vi "log analysis_gps.vi"() -> ()   [LabVIEW 2019] (continued)
,0.3081,0.6694,0.1254,0.0948,0.0826,0.1629,0.1651,5.0479,0f000001,0*dfc03d63\n\t", "INSPVAXA,USB3,0,48.5,FINESTEERING,2107,281764.150,02000000,471d,15824;INS_ALIGNMENT_COMPLETE,INS_RTKFIXED,37.37122080817,126.72272865797,8.0273,22.3000,-0.0183,0.2610,0.0199,-0.883754251,-0.497263643,91.594297223,0.5508,0.3085,0.6797,0.1258,0.0948,0.0829,0.1629,0.1651,5.0491,0f000001,0*98c9c36a\n\t", "INSPVAXA,USB3,0,48.5,FINESTEERING,2107,281764.650,02000000,471d,15824;INS_ALIGNMENT_COMPLETE,INS_RTKFIXED,37.37122075325,126.72273024996,8.0307,22.3000,-0.0230,0.2873,0.0155,-0.910536369,-0.571169391,91.698573448,0.5508,0.3085,0.6797,0.1258,0.0948,0.0829,0.1629,0.1651,5.0491,0f000001,0*a48c0ed7\n\t", "INSPVAXA,USB3,0,49.5,FINESTEERING,2107,281765.150,02000000,471d,15824;INS_ALIGNMENT_COMPLETE,INS_RTKFIXED,37.37122068841,126.72273183543,8.0343,22.3000,-0.0165,0.2820,0.0133,-0.835088790,-0.555071717,91.791979713,0.5558,0.3086,0.6882,0.1257,0.0948,0.0832,0.1628,0.1650,5.0496,0f000001,0*cba52910\n\t", "INSPVAXA,USB3,0,49.5,FINESTEERING,2107,281765.650,02000000,471d,15824;INS_ALIGNMENT_COMPLETE,INS_RTKFIXED,37.37122061486,126.72273346284,8.0365,22.3000,-0.0171,0.2746,0.0152,-0.832834423,-0.571575823,91.924169920,0.5558,0.3086,0.6882,0.1257,0.0948,0.0832,0.1628,0.1650,5.0496,0f000001,0*526b2e24\n\t", "INSPVAXA,USB3,0,49.0,FINESTEERING,2107,281766.150,02000000,471d,15824;INS_ALIGNMENT_COMPLETE,INS_RTKFIXED,37.37122054097,126.72273507488,8.0385,22.3000,-0.0218,0.2706,0.0128,-1.000637631,-0.672076774,92.055365430,0.5592,0.3087,0.6949,0.1259,0.0948,0.0833,0.1628,0.1650,5.0498,0f000001,0*57bf3361\n\t", "INSPVAXA,USB3,0,49.0,FINESTEERING,2107,281766.650,02000000,471d,15824;INS_ALIGNMENT_COMPLETE,INS_RTKFIXED,37.37122044479,126.72273670968,8.0412,22.3000,-0.0285,0.2846,0.0116,-1.092573740,-0.740242490,92.171373793,0.5592,0.3087,0.6949,0.1259,0.0948,0.0833,0.1628,0.1650,5.0498,0f000001,0*1c223ea9\n\t", "INSPVAXA,USB3,0,48.0,FINESTEERING,2107,281767.150,02000000,471d,15824;INS_ALIGNMENT_COMPLETE,INS_RTKFIXED,37.37122033445,126.72273829026,8.0449,22.3000,-0.0305,0.2613,0.0217,-0.977094539,-0.639903649,92.271203612,0.5614,0.3086,0.7003,0.1258,0.0947,0.0834,0.1628,0.1649,5.0495,0f000001,0*5c3b8fb1\n\t", "INSPVAXA,USB3,0,48.0,FINESTEERING,2107,281767.650,02000000,471d,15824;INS_ALIGNMENT_COMPLETE,INS_RTKFIXED,37.37122021827,126.72273994335,8.0476,22.3000,-0.0288,0.2733,0.0197,-0.964628632,-0.656119186,92.463441538,0.5614,0.3086,0.7003,0.1258,0.0947,0.0834,0.1628,0.1649,5.0495,0f000001,0*cc7927eb\n\t", "INSPVAXA,USB3,0,48.0,FINESTEERING,2107,281768.150,02000000,471d,15824;INS_ALIGNMENT_COMPLETE,INS_RTKFIXED,37.37122009872,126.72274157958,8.0500,22.3000,-0.0294,0.2847,0.0191,-0.946431620,-0.566462229,92.660906936,0.5627,0.3085,0.7043,0.1259,0.0947,0.0835,0.1628,0.1649,5.0496,0f000001,0*cc13fb9d\n\t", "INSPVAXA,USB3,0,49.0,FINESTEERING,2107,281768.650,02000000,471d,15824;INS_ALIGNMENT_COMPLETE,INS_RTKFIXED,37.37121997801,126.72274320142,8.0509,22.3000,-0.0214,0.2856,0.0260,-1.015543433,-0.231279609,92.847402266,0.5627,0.3085,0.7043,0.1259,0.0947,0.0835,0.1628,0.1649,5.0496,0f000001,0*22053697\n\t", "INSPVAXA,USB3,0,46.5,FINESTEERING,2107,281769.650,02000000,471d,15824;INS_ALIGNMENT_COMPLETE,INS_RTKFIXED,37.37121967893,126.72274645196,8.0567,22.3000,-0.0370,0.2793,0.0333,-0.818626182,0.216920532,93.214992796,0.5635,0.3085,0.7075,0.1258,0.0947,0.0835,0.1628,0.1649,5.0499,0f000001,0*792e5a9d\n\t", "INSPVAXA,USB3,0,48.5,FINESTEERING,2107,281771.150,02000000,471d,15824;INS_ALIGNMENT_COMPLETE,INS_RTKFIXED,37.37121916335,126.72275134411,8.0669,22.3000,-0.0460,0.2833,0.0183,-0.792418480,0.032350312,93.864070762,0.5648,0.3085,0.7116,0.1262,0.0947,0.0836,0.1628,0.1649,5.0523,0f000001,0*03020e62\n\t", "INSPVAXA,USB3,0,47.0,FINESTEERING,2107,281772.150,02000000,471d,15824;INS_ALIGNMENT_COMPLETE,INS_RTKFIXED,37.37121879734,126.72275457125,8.0729,22.3000,-0.0562,0.2927,0.0149,-0.701118394,-0.215535385,94.262257179,0.5652,0.3086,0.7131,0.1264,0.0948,0.0837,0.1628,0.1649,5.0539,0f000001,0*6742cf9b\n\t", "INSPVAXA,USB3,0,47.5,FINESTEERING,2107,281773.150,02000000,471d,15824;INS_ALIGNMENT_COMPLETE,INS_RTKFIXED,37.37121842061,126.72275777876,8.0764,22.3000,-0.0402,0.2880,0.0117,-0.782099339,-0.380092330,94.588227053,0.5655,0.3117,0.7220,0.1266,0.0954,0.0843,0.1628,0.1649,5.0554,0f000001,0*2c781ada\n\t", "INSPVAXA,USB3,0,47.5,FINESTEERING,2107,281774.650,02000000,471d,15824;INS_ALIGNMENT_COMPLETE,INS_RTKFIXED,37.37121790104,126.72276172821,8.0844,22.3000,-0.0056,-0.1159,0.0265,-0.829469010,-1.054819962,94.805665616,0.5657,0.3125,0.7262,0.1269,0.0954,0.0845,0.1628,0.1649,5.0568,0f000001,0*5083390f\n\t", "INSPVAXA,USB3,0,45.5,FINESTEERING,2107,281775.650,02000000,471d,15824;INS_ALIGNMENT_COMPLETE,INS_RTKFIXED,37.37121775993,126.72276174880,8.0908,22.3000,-0.0341,0.2302,0.0228,-0.820870768,-0.784541706,94.618919565,0.5657,0.3121,0.7276,0.1285,0.0952,0.0845,0.1627,0.1649,5.0580,0f000001,0*ef5961e6\n\t", "INSPVAXA,USB3,0,49.5,FINESTEERING,2107,281777.150,02000000,471d,15824;INS_ALIGNMENT_COMPLETE,INS_RTKFIXED,37.37121742515,126.72276471335,8.0933,22.3000,-0.0434,0.3635,0.0199,-0.788823341,-1.034155621,94.704274658,0.5667,0.3105,0.7263,0.1288,0.0950,0.0844,0.1627,0.1648,5.0605,0f000001,0*58cfd0fe\n\t", "INSPVAXA,USB3,0,49.5,FINESTEERING,2107,281780.650,02000000,471d,15824;INS_ALIGNMENT_COMPLETE,INS_RTKFIXED,37.37121639807,126.72277573033,8.0654,22.3000,-0.0075,0.2871,0.0244,-0.701767133,-0.824742936,91.476878975,0.4298,0.3000,0.6003,0.1163,0.0939,0.0789,0.1625,0.1636,5.0634,0f000001,0*3e81e8f3\n\t", "INSPVAXA,USB3,0,49.0,FINESTEERING,2107,281782.150,02000000,471d,15824;INS_ALIGNMENT_COMPLETE,INS_RTKFIXED,37.37121614895,126.72278060077,8.0494,22.3000,-0.0125,0.2941,0.0170,-0.958151284,-0.907972358,90.050842278,0.4192,0.2995,0.5761,0.1162,0.0938,0.0788,0.1624,0.1635,5.0656,0f000001,0*79d70d48\n\t", "INSPVAXA,USB3,0,48.0,FINESTEERING,2107,281794.200,02000000,471d,15824;INS_ALIGNMENT_COMPLETE,INS_RTKFIXED,37.37121538500,126.72279353221,7.9323,22.3000,0.0019,0.0033,0.0055,-1.472038191,-1.222257427,90.266116104,0.2743,0.1995,0.4008,0.0352,0.0349,0.0325,0.1516,0.1495,5.0388,0f000005,0*12f5b6da\n\t", "INSPVAXA,USB3,0,48.0,FINESTEERING,2107,281796.200,02000000,471d,15824;INS_ALIGNMENT_COMPLETE,INS_RTKFIXED,37.37121541125,126.72279352515,7.9254,22.3000,-0.0002,0.0035,0.0060,-1.463145311,-1.218768654,90.268956721,0.2548,0.1854,0.3737,0.0345,0.0343,0.0314,0.1516,0.1493,5.0350,0f000005,0*63f626df\n\t", "INSPVAXA,USB3,0,43.0,FINESTEERING,2107,281797.700,02000000,471d,15824;INS_ALIGNMENT_COMPLETE,INS_RTKFIXED,37.37121541556,126.72279591257,7.9222,22.3000,-0.0052,0.3417,0.0085,-1.766936692,-1.171645490,90.396175106,0.2469,0.1802,0.3627,0.0345,0.0343,0.0313,0.1515,0.1492,5.0303,0f000005,0*2970234a\n\t", "INSPVAXA,USB3,0,45.5,FINESTEERING,2107,281798.700,02000000,471d,15824;INS_ALIGNMENT_COMPLETE,INS_RTKFIXED,37.37121535057,126.72279879079,7.9235,22.3000,-0.0085,0.3000,0.0138,-1.696631834,-1.054944377,90.699133923,0.2423,0.1802,0.3574,0.0527,0.0471,0.0400,0.1536,0.1513,5.0319,0f000001,0*b28cf3b5\n\t", "INSPVAXA,USB3,0,46.0,FINESTEERING,2107,281800.200,02000000,471d,15824;INS_ALIGNMENT_COMPLETE,INS_RTKFIXED,37.37121518346,126.72280384244,7.9320,22.3000,-0.0138,0.3041,-0.0020,-1.831014383,-0.921017115,91.358421751,0.2498,0.2023,0.3609,0.0772,0.0698,0.0531,0.1576,0.1555,5.0235,0f000001,0*fd249ab4\n\t", "INSPVAXA,USB3,0,45.0,FINESTEERING,2107,281801.700,02008000,471d,15824;INS_ALIGNMENT_COMPLETE,INS_RTKFIXED,37.37121487597,126.72280876147,7.9415,22.3000,-0.0281,0.2809,0.0050,-1.870107911,-0.684128774,92.617548886,0.2701,0.2229,0.3702,0.0875,0.0787,0.0583,0.1591,0.1573,5.0044,0f000001,0*b89165ad\n\t", "INSPVAXA,USB3,0,48.0,FINESTEERING,2107,281802.700,02008000,471d,15824;INS_ALIGNMENT_COMPLETE,INS_RTKFIXED,37.37121453908,126.72281198538,7.9511,22.3000,-0.0315,0.2792,0.0111,-1.788436181,-0.484915836,93.932977011,0.2978,0.2449,0.3840,0.0951,0.0852,0.0628,0.1602,0.1589,4.9745,0f000001,0*1b429bef\n\t", "INSPVAXA,USB3,0,48.5,FINESTEERING,2107,281804.200,02008000,471d,15824;INS_ALIGNMENT_COMPLETE,INS_RTKFIXED,37.37121383035,126.72281674518,7.9651,22.3000,-0.0315,0.2774,0.0174,-1.651879586,-0.284385340,95.400888665,0.3536,0.2781,0.4212,0.1050,0.0912,0.0696,0.1611,0.1606,4.9104,0f000001,0*27f05722\n\t", "INSPVAXA,USB3,0,48.5,FINESTEERING,2107,281804.700,02008000,471d,15824;INS_ALIGNMENT_COMPLETE,INS_RTKFIXED,37.37121355118,126.72281832287,7.9691,22.3000,-0.0490,0.2623,0.0114,-1.600367868,-0.284854057,95.675635132,0.3536,0.2781,0.4212,0.1050,0.0912,0.0696,0.1611,0.1606,4.9104,0f000001,0*fdce50cc\n\t", "INSPVAXA,USB3,0,47.5,FINESTEERING,2107,281806.200,02000000,471d,15824;INS_ALIGNMENT_COMPLETE,INS_RTKFIXED,37.37121269576,126.72282281458,7.9853,22.3000,-0.0549,0.2699,0.0235,-1.099815041,-0.190468307,96.163961880,0.3893,0.2926,0.4618,0.1082,0.0921,0.0739,0.1610,0.1610,4.8764,0f000001,0*3796a6d3\n\t", "INSPVAXA,USB3,0,49.0,FINESTEERING,2107,281807.200,02000000,471d,15824;INS_ALIGNMENT_COMPLETE,INS_RTKFIXED,37.37121211278,126.72282605036,7.9969,22.3000,-0.0568,0.3027,0.0138,-1.053067803,-0.177291074,96.270087858,0.3995,0.2955,0.4805,0.1085,0.0920,0.0753,0.1609,0.1610,4.8712,0f000001,0*6bce3c8a\n\t", "INSPVAXA,USB3,0,49.0,FINESTEERING,2107,281807.700,02000000,471d,15824;INS_ALIGNMENT_COMPLETE,INS_RTKFIXED,37.37121182995,126.72282768938,8.0018,22.3000,-0.0581,0.2574,0.0176,-1.058374656,-0.238658340,96.102791514,0.3995,0.2955,0.4805,0.1085,0.0920,0.0753,0.1609,0.1610,4.8712,0f000001,0*be10ea19\n\t", "INSPVAXA,USB3,0,50.0,FINESTEERING,2107,281808.200,02000000,471d,15824;INS_ALIGNMENT_COMPLETE,INS_RTKFIXED,37.37121156109,126.72282925658,8.0066,22.3000,-0.0729,0.2643,0.0186,-0.872363263,-0.172820983,95.527165768,0.4058,0.2969,0.4970,0.1085,0.0920,0.0762,0.1608,0.1609,4.8702,0f000001,0*2e1aa4d5\n\t", "INSPVAXA,USB3,0,47.5,FINESTEERING,2107,281810.700,02000000,471d,15824;INS_ALIGNMENT_COMPLETE,INS_RTKFIXED,37.37121067103,126.72283703860,8.0191,22.3000,-0.0356,0.2756,0.0276,-0.647693750,-0.582187036,89.865016518,0.4124,0.2979,0.5229,0.1081,0.0920,0.0770,0.1607,0.1609,4.8726,0f000001,0*855b65fe\n\t", "INSPVAXA,USB3,0,45.5,FINESTEERING,2107,281811.200,02000000,471d,15824;INS_ALIGNMENT_COMPLETE,INS_RTKFIXED,37.37121058449,126.72283863071,8.0196,22.3000,-0.0335,0.2776,0.0134,-0.642436462,-0.620062849,88.791539404,0.4132,0.2980,0.5319,0.1079,0.0921,0.0771,0.1607,0.1609,4.8738,0f000001,0*5d2242c7\n\t", "INSPVAXA,USB3,0,45.5,FINESTEERING,2107,281811.700,02000000,471d,15824;INS_ALIGNMENT_COMPLETE,INS_RTKFIXED,37.37121052303,126.72284024830,8.0190,22.3000,-0.0385,0.2808,0.0125,-0.613070377,-0.534497293,88.053265281,0.4132,0.2980,0.5319,0.1079,0.0921,0.0771,0.1607,0.1609,4.8738,0f000001,0*21e07958\n\t", "INSPVAXA,USB3,0,48.5,FINESTEERING,2107,281812.200,02000000,471d,15824;INS_ALIGNMENT_COMPLETE,INS_RTKFIXED,37.37121047493,126.72284184822,8.0183,22.3000,-0.0314,0.2883,0.0148,-0.539418931,-0.410155130,87.563487932,0.4135,0.2980,0.5387,0.1083,0.0923,0.0770,0.1607,0.1609,4.8744,0f000001,0*aee609c3\n\t", "INSPVAXA,USB3,0,48.5,FINESTEERING,2107,281812.700,02000000,471d,15824;INS_ALIGNMENT_COMPLETE,INS_RTKFIXED,37.37121044769,126.72284347413,8.0176,22.3000,-0.0247,0.2718,0.0203,-0.569551057,-0.519035178,87.323829382,0.4135,0.2980,0.5387,0.1083,0.0923,0.0770,0.1607,0.1609,4.8744,0f000001,0*0b29fab3\n\t", "INSPVAXA,USB3,0,49.5,FINESTEERING,2107,281813.200,02000000,471d,15824;INS_ALIGNMENT_COMPLETE,INS_RTKFIXED,37.37121043009,126.72284509802,8.0163,22.3000,-0.0270,0.2716,0.0250,-0.708149800,-0.786508619,87.284677212,0.4137,0.2982,0.5437,0.1082,0.0926,0.0769,0.1607,0.1609,4.8743,0f000001,0*3e525f31\n\t", "INSPVAXA,USB3,0,49.5,FINESTEERING,2107,281813.700,02000000,471d,15824;INS_ALIGNMENT_COMPLETE,INS_RTKFIXED,37.37121041419,126.72284671710,8.0139,22.3000,-0.0269,0.2730,0.0206,-0.734434421,-0.847262919,87.384621044,0.4137,0.2982,0.5437,0.1082,0.0926,0.0769,0.1607,0.1609,4.8743,0f000001,0*ad1d52fd\n\t", "INSPVAXA,USB3,0,51.5,FINESTEERING,2107,281814.200,02000000,471d,15824;INS_ALIGNMENT_COMPLETE,INS_RTKFIXED,37.37121039679,126.72284831835,8.0121,22.3000,-0.0282,0.2780,0.0157,-0.723695017,-0.718771223,87.478292195,0.4133,0.2982,0.5471,0.1087,0.0929,0.0768,0.1607,0.1609,4.8744,0f000001,0*2471b93a\n\t", "INSPVAXA,USB3,0,51.5,FINESTEERING,2107,281814.700,02000000,471d,15824;INS_ALIGNMENT_COMPLETE,INS_RTKFIXED,37.37121037596,126.72284994702,8.0093,22.3000,-0.0392,0.2745,0.0084,-0.653618450,-0.794919707,87.628354192,0.4133,0.2982,0.5471,0.1087,0.0929,0.0768,0.1607,0.1609,4.8744,0f000001,0*e403a187\n\t", "INSPVAXA,USB3,0,48.5,FINESTEERING,2107,281815.200,02000000,471d,15824;INS_ALIGNMENT_COMPLETE,INS_RTKFIXED,37.37121035462,126.72285153134,8.0061,22.3000,-0.0298,0.2645,0.0056,-0.689462144,-0.765571273,87.819585359,0.4135,0.2983,0.5496,0.1092,0.0931,0.0767,0.1607,0.1609,4.8745,0f000001,0*3d6e9c36\n\t", "INSPVAXA,USB3,0,48.5,FINESTEERING,2107,281815.700,02000000,471d,15824;INS_ALIGNMENT_COMPLETE,INS_RTKFIXED,37.37121033500,126.72285311005,8.0032,22.3000,-0.0264,0.2987,0.0158,-0.781716650,-0.583090906,88.033249941,0.4135,0.2983,0.5496,0.1092,0.0931,0.0767,0.1607,0.1609,4.8745,0f000001,0*4dfcf1d6\n\t", "INSPVAXA,USB3,0,51.0,FINESTEERING,2107,281816.200,02008000,471d,15824;INS_ALIGNMENT_COMPLETE,INS_RTKFIXED,37.37121030517,126.72285487145,8.0002,22.3000,-0.0425,0.2860,0.0120,-0.722434536,-0.707507472,88.283028579,0.4136,0.2984,0.5510,0.1094,0.0933,0.0766,0.1607,0.1609,4.8747,0f000001,0*7939fe65\n\t", "INSPVAXA,USB3,0,51.0,FINESTEERING,2107,281816.700,02008000,471d,15824;INS_ALIGNMENT_COMPLETE,INS_RTKFIXED,37.37121027801,126.72285655609,7.9980,22.3000,-0.0398,0.3098,0.0245,-0.754705884,-0.828367575,88.621683950,0.4136,0.2984,0.5510,0.1094,0.0933,0.0766,0.1607,0.1609,4.8747,0f000001,0*590aa229\n\t", "INSPVAXA,USB3,0,48.5,FINESTEERING,2107,281817.200,02008000,471d,15824;INS_ALIGNMENT_COMPLETE,INS_RTKFIXED,37.37121021919,126.72285821539,7.9935,22.3000,-0.0399,0.3049,0.0009,-0.558805216,-0.866819508,89.180337786,0.4133,0.2986,0.5518,0.1098,0.0934,0.0766,0.1606,0.1608,4.8755,0f000001,0*c032cfc0\n\t", "INSPVAXA,USB3,0,48.5,FINESTEERING,2107,281817.700,02008000,471d,15824;INS_ALIGNMENT_COMPLETE,INS_RTKFIXED,37.37121014797,126.72285990079,7.9875,22.3000,-0.0366,0.2866,-0.0014,-0.542824992,-1.209169915,90.078081458,0.4133,0.2986,0.5518,0.1098,0.0934,0.0766,0.1606,0.1608,4.8755,0f000001,0*9b0194b0\n\t", "INSPVAXA,USB3,0,48.0,FINESTEERING,2107,281818.200,02008000,471d,15824;INS_ALIGNMENT_COMPLETE,INS_RTKFIXED,37.37121006905,126.72286154850,7.9830,22.3000,-0.0357,0.2838,0.0134,-0.818598247,-1.286018630,91.179102857,0.4133,0.2987,0.5521,0.1099,0.0933,0.0766,0.1606,0.1607,4.8765,0f000001,0*fb948376\n\t", "INSPVAXA,USB3,0,48.0,FINESTEERING,2107,281818.700,02008000,471d,15824;INS_ALIGNMENT_COMPLETE,INS_RTKFIXED,37.37120996329,126.72286319027,7.9792,22.3000,-0.0377,0.2984,0.0070,-0.940731055,-1.250722578,92.396481410,0.4133,0.2987,0.5521,0.1099,0.0933,0.0766,0.1606,0.1607,4.8765,0f000001,0*0f67b83c\n\t", "INSPVAXA,USB3,0,49.0,FINESTEERING,2107,281819.200,02008000,471d,15824;INS_ALIGNMENT_COMPLETE,INS_RTKFIXED,37.37120981052,126.72286484515,7.9750,22.3000,-0.0478,0.2879,0.0099,-0.798984239,-1.444181950,93.568970081,0.4129,0.2987,0.5522,0.1099,0.0932,0.0766,0.1605,0.1605,4.8778,0f000001,0*6b031fe9\n\t", "INSPVAXA,USB3,0,49.0,FINESTEERING,2107,281819.700,02008000,471d,15824;INS_ALIGNMENT_COMPLETE,INS_RTKFIXED,37.37120962300,126.72286650676,7.9705,22.3000,-0.0671,0.2946,0.0135,-0.649128294,-1.472904568,94.664078192,0.4129,0.2987,0.5522,0.1099,0.0932,0.0766,0.1605,0.1605,4.8778,0f000001,0*2bf58c7b\n\t", "INSPVAXA,USB3,0,48.5,FINESTEERING,2107,281820.200,02008000,471d,15824;INS_ALIGNMENT_COMPLETE,INS_RTKFIXED,37.37120940139,126.72286814747,7.9651,22.3000,-0.0641,0.2873,0.0149,-0.504838875,-1.441095327,95.746291084,0.4127,0.2987,0.5521,0.1098,0.0930,0.0766,0.1605,0.1604,4.8792,0f000001,0*7c1d55f3\n\t", "INSPVAXA,USB3,0,48.5,FINESTEERING,2107,281820.700,02008000,471d,15824;INS_ALIGNMENT_COMPLETE,INS_RTKFIXED,37.37120917103,126.72286978921,7.9589,22.3000,-0.0688,0.2879,0.0058,-0.603273984,-1.593663516,96.633630255,0.4127,0.2987,0.5521,0.1098,0.0930,0.0766,0.1605,0.1604,4.8792,0f000001,0*e21ec5f9\n\t", "DUALANTENNAHEADINGA,USB3,0,48.5,FINESTEERING,2107,281821.200,02000000,d426,15824;SOL_COMPUTED,NARROW_FLOAT,-1.000000000,199.802429199,59.611751556,0.0,103.871536255,169.545913696,\"631T\",19,8,8,8,04,00,20,23*e0db817a\n\t", "INSPVAXA,USB3,0,48.5,FINESTEERING,2107,281821.700,02000000,471d,15824;INS_ALIGNMENT_COMPLETE,INS_RTKFIXED,37.37120867107,126.72287305353,7.9486,22.3000,-0.0854,0.2737,-0.0020,-0.718036711,-1.580500229,97.593601208,0.4126,0.2986,0.5520,0.1098,0.0929,0.0766,0.1604,0.1603,4.8804,0f000001,0*a82ce81c\n\t", "INSPVAXA,USB3,0,51.0,FINESTEERING,2107,281822.200,02000000,471d,15824;INS_ALIGNMENT_COMPLETE,INS_RTKFIXED,37.37120839710,126.72287464148,7.9433,22.3000,-0.0737,0.2706,0.0058,-0.493099711,-1.491040971,97.883869188,0.4123,0.2985,0.5518,0.1098,0.0930,0.0767,0.1604,0.1602,4.8814,0f000001,0*43cf4a7f\n\t", "DUALANTENNAHEADINGA,USB3,0,51.0,FINESTEERING,2107,281822.700,02000000,d426,15824;SOL_COMPUTED,NARROW_FLOAT,-1.000000000,199.656448364,63.340484619,0.0,99.066596985,82.183616638,\"631T\",18,8,8,8,04,00,20,23*3eb0b03b\n\t", "INSPVAXA,USB3,0,46.0,FINESTEERING,2107,281823.200,02000000,471d,15824;INS_ALIGNMENT_COMPLETE,INS_RTKFIXED,37.37120785592,126.72287776108,7.9348,22.3000,-0.0813,0.2968,0.0005,-0.426101177,-1.082566624,98.131503900,0.4122,0.2985,0.5517,0.1098,0.0931,0.0768,0.1603,0.1602,4.8821,0f000001,0*e97d0866\n\t", "DUALANTENNAHEADINGA,USB3,0,46.0,FINESTEERING,2107,281823.700,02000000,d426,15824;SOL_COMPUTED,NARROW_FLOAT,-1.000000000,152.081710815,66.315963745,0.0,360.000000000,174.707107544,\"631T\",18,9,9,8,04,00,20,23*2d86097d\n\t", "DUALANTENNAHEADINGA,USB3,0,50.0,FINESTEERING,2107,281824.200,02000000,d426,15824;SOL_COMPUTED,NARROW_FLOAT,-1.000000000,155.447463989,72.039955139,0.0,360.000000000,145.525100708,\"631T\",18,9,9,8,04,00,20,23*f6d7a9cd\n\t", "INSPVAXA,USB3,0,50.0,FINESTEERING,2107,281824.700,02000000,471d,15824;INS_ALIGNMENT_COMPLETE,INS_RTKFIXED,37.37120702523,126.72288248256,7.9286,22.3000,-0.1000,0.2970,-0.0030,-0.414363931,-1.319109492,98.317764432,0.4124,0.2984,0.5515,0.1099,0.0933,0.0768,0.1603,0.1602,4.8829,0f000001,0*6aa4622c\n\t", "DUALANTENNAHEADINGA,USB3,0,49.5,FINESTEERING,2107,281825.200,02000000,d426,15824;SOL_COMPUTED,L1_FLOAT,-1.000000000,69.256408691,12.160554886,0.0,285.962799072,180.000000000,\"631T\",19,8,8,5,04,00,20,21*0683b703\n\t", "INSPVAXA,USB3,0,49.5,FINESTEERING,2107,281825.700,02000000,471d,15824;INS_ALIGNMENT_COMPLETE,INS_RTKFIXED,37.37120646463,126.72288578375,7.9281,22.3000,-0.0763,0.2904,0.0216,-0.793323324,-0.889298592,98.320200190,0.4125,0.2985,0.5514,0.1101,0.0934,0.0769,0.1602,0.1602,4.8839,0f000001,0*5f866581\n\t", "INSPVAXA,USB3,0,48.5,FINESTEERING,2107,281826.200,02000000,471d,15824;INS_ALIGNMENT_COMPLETE,INS_RTKFIXED,37.37120619057,126.72288730405,7.9253,22.3000,-0.0749,0.2848,0.0194,-0.697963338,-0.472482314,97.902378657,0.4129,0.2985,0.5514,0.1102,0.0935,0.0770,0.1601,0.1601,4.8852,0f000001,0*4b4d602c\n\t", "INSPVAXA,USB3,0,48.5,FINESTEERING,2107,281826.700,02000000,471d,15824;INS_ALIGNMENT_COMPLETE,INS_RTKFIXED,37.37120593844,126.72288885558,7.9222,22.3000,-0.0660,0.2989,0.0157,-0.925431746,0.038687863,97.361199599,0.4129,0.2985,0.5514,0.1102,0.0935,0.0770,0.1601,0.1601,4.8852,0f000001,0*d022d5ea\n\t", "DUALANTENNAHEADINGA,USB3,0,49.5,FINESTEERING,2107,281827.200,02000000,d426,15824;SOL_COMPUTED,NARROW_FLOAT,-1.000000000,106.272483826,69.863449097,0.0,360.000000000,180.000000000,\"631T\",18,5,5,5,04,00,20,03*ec53100b\n\t", "INSPVAXA,USB3,0,49.5,FINESTEERING,2107,281827.700,02000000,471d,15824;INS_ALIGNMENT_COMPLETE,INS_RTKFIXED,37.37120552459,126.72289199783,7.9230,22.3000,-0.0613,0.2731,0.0106,-1.441869650,0.390097771,95.831538133,0.4135,0.2986,0.5515,0.1109,0.0937,0.0770,0.1599,0.1601,4.8868,0f000001,0*586a71ed\n\t", "INSPVAXA,USB3,0,51.0,FINESTEERING,2107,281828.200,02000000,471d,15824;INS_ALIGNMENT_COMPLETE,INS_RTKFIXED,37.37120533257,126.72289355096,7.9234,22.3000,-0.0675,0.2814,0.0290,-1.476207155,0.673066178,94.890255810,0.4144,0.2985,0.5514,0.1108,0.0941,0.0770,0.1598,0.1600,4.8875,0f000001,0*65bdbb94\n\t", "INSPVAXA,USB3,0,51.0,FINESTEERING,2107,281828.700,02000000,471d,15824;INS_ALIGNMENT_COMPLETE,INS_RTKFIXED,37.37120515804,126.72289518020,7.9256,22.3000,-0.0694,0.2933,0.0211,-1.265355938,0.544212560,94.152212733,0.4144,0.2985,0.5514,0.1108,0.0941,0.0770,0.1598,0.1600,4.8875,0f000001,0*3fa45f89\n\t", "INSPVAXA,USB3,0,46.5,FINESTEERING,2107,281829.200,02000000,471d,15824;INS_ALIGNMENT_COMPLETE,INS_RTKFIXED,37.37120502580,126.72289678148,7.9278,22.3000,-0.0502,0.2768,0.0145,-1.429978780,0.528599128,93.605134571,0.4154,0.2985,0.5516,0.1105,0.0939,0.0771,0.1597,0.1599,4.8857,0f000001,0*990165b1\n\t", "DUALANTENNAHEADINGA,USB3,0,46.5,FINESTEERING,2107,281829.700,02000000,d426,15824;SOL_COMPUTED,NARROW_FLOAT,-1.000000000,57.886253357,2.555429220,0.0,154.963073730,180.000000000,\"631T\",19,7,7,5,04,00,20,03*f9e0cff3\n\t", "DUALANTENNAHEADINGA,USB3,0,49.5,FINESTEERING,2107,281830.200,02000000,d426,15824;SOL_COMPUTED,L1_FLOAT,-1.000000000,83.986137390,10.132819176,0.0,360.000000000,180.000000000,\"631T\",19,6,6,3,04,00,20,01*1abfa712\n\t", "INSPVAXA,USB3,0,49.5,FINESTEERING,2107,281830.700,02000000,471d,15824;INS_ALIGNMENT_COMPLETE,INS_RTKFIXED,37.37120465229,126.72290157166,7.9350,22.3000,-0.0442,0.2947,0.0242,-1.334244960,0.390910805,92.567102853,0.4155,0.2984,0.5517,0.1101,0.0937,0.0771,0.1595,0.1599,4.8819,0f000001,0*e118fdc5\n\t", "DUALANTENNAHEADINGA,USB3,0,50.0,FINESTEERING,2107,281831.200,02000000,d426,15824;SOL_COMPUTED,NARROW_FLOAT,-1.000000000,59.043685913,-28.864562988,0.0,170.366668701,180.000000000,\"631T\",18,8,8,7,04,00,20,23*14dad2b0\n\t", "DUALANTENNAHEADINGA,USB3,0,50.0,FINESTEERING,2107,281831.700,02000000,d426,15824;SOL_COMPUTED,NARROW_FLOAT,-1.000000000,59.094017029,-28.251525879,0.0,171.144256592,180.000000000,\"631T\",17,8,8,7,04,00,20,23*b1c96c44\n\t", "DUALANTENNAHEADINGA,USB3,0,51.0,FINESTEERING,2107,281832.200,02000000,d426,15824;SOL_COMPUTED,NARROW_FLOAT,-1.000000000,147.351470947,72.022521973,0.0,360.000000000,180.000000000,\"631T\",17,7,7,7,04,00,20,23*e605d7f3\n\t", "DUALANTENNAHEADINGA,USB3,0,51.0,FINESTEERING,2107,281832.700,02000000,d426,15824;SOL_COMPUTED,NARROW_FLOAT,-1.000000000,140.025573730,68.472808838,0.0,360.000000000,180.000000000,\"631T\",16,7,7,7,04,00,20,23*882fbccd\n\t", "DUALANTENNAHEADINGA,USB3,0,50.5,FINESTEERING,2107,281833.200,02000000,d426,15824;SOL_COMPUTED,NARROW_FLOAT,-1.000000000,68.082496643,-11.763427734,0.0,169.499374390,180.000000000,\"631T\",18,9,9,7,04,00,20,23*031ca633\n\t", "DUALANTENNAHEADINGA,USB3,0,50.5,FINESTEERING,2107,281833.700,02000000,d426,15824;SOL_COMPUTED,NARROW_FLOAT,-1.000000000,67.931724548,-11.679229736,0.0,169.789916992,180.000000000,\"631T\",18,9,9,7,04,00,20,23*9183d900\n\t", "DUALANTENNAHEADINGA,USB3,0,47.0,FINESTEERING,2107,281834.200,02000000,d426,15824;SOL_COMPUTED,NARROW_FLOAT,-1.000000000,117.470924377,63.855136871,0.0,360.000000000,180.000000000,\"631T\",18,5,5,5,04,00,20,03*04244261\n\t", "INSPVAXA,USB3,0,47.0,FINESTEERING,2107,281834.700,02000000,471d,15824;INS_ALIGNMENT_COMPLETE,INS_RTKFIXED,37.37120376020,126.72291436834,7.9622,22.3000,-0.0339,0.2802,0.0380,-1.719157085,0.362405119,93.876835430,0.4140,0.2983,0.5521,0.1098,0.0930,0.0772,0.1595,0.1599,4.8699,0f000001,0*4c3c706d\n\t", "DUALANTENNAHEADINGA,USB3,0,49.5,FINESTEERING,2107,281835.200,02000000,d426,15824;SOL_COMPUTED,NARROW_FLOAT,-1.000000000,56.406482697,-13.603881836,0.0,133.707977295,180.000000000,\"631T\",17,6,6,5,04,00,20,03*0c459025\n\t", "DUALANTENNAHEADINGA,USB3,0,49.5,FINESTEERING,2107,281835.700,02000000,d426,15824;SOL_COMPUTED,NARROW_FLOAT,-1.000000000,56.377288818,-12.403900146,0.0,134.026809692,180.000000000,\"631T\",18,6,6,5,04,00,20,03*a9390bed\n\t", "INSPVAXA,USB3,0,49.5,FINESTEERING,2107,281836.200,02000000,471d,15824;INS_ALIGNMENT_COMPLETE,INS_RTKFIXED,37.37120330531,126.72291919762,7.9715,22.3000,-0.0485,0.2910,0.0305,-1.607227145,0.177759790,96.248616069,0.4130,0.2982,0.5522,0.1099,0.0930,0.0773,0.1596,0.1599,4.8709,0f000001,0*7239ccf3\n\t", "DUALANTENNAHEADINGA,USB3,0,49.5,FINESTEERING,2107,281836.700,02000000,d426,15824;SOL_COMPUTED,L1_FLOAT,-1.000000000,75.942611694,16.211278915,0.0,339.522399902,180.000000000,\"631T\",19,6,6,3,04,00,20,01*51b3f26e\n\t", "DUALANTENNAHEADINGA,USB3,0,48.5,FINESTEERING,2107,281837.200,02000000,d426,15824;SOL_COMPUTED,L1_FLOAT,-1.000000000,80.771942139,6.980556488,0.0,360.000000000,180.000000000,\"631T\",20,5,5,2,04,00,20,01*7f238ca7\n\t", "DUALANTENNAHEADINGA,USB3,0,48.5,FINESTEERING,2107,281837.700,02000000,d426,15824;SOL_COMPUTED,L1_FLOAT,-1.000000000,81.947074890,7.586090088,0.0,360.000000000,180.000000000,\"631T\",19,5,5,2,04,00,20,01*fab92539\n\t", "DUALANTENNAHEADINGA,USB3,0,50.5,FINESTEERING,2107,281838.200,02000000,d426,15824;SOL_COMPUTED,NARROW_FLOAT,-1.000000000,70.339691162,-8.337524414,0.0,360.000000000,180.000000000,\"631T\",19,5,5,5,04,00,20,03*774b3c80\n\t", "DUALANTENNAHEADINGA,USB3,0,50.5,FINESTEERING,2107,281838.700,02000000,d426,15824;SOL_COMPUTED,NARROW_FLOAT,-1.000000000,76.530433655,10.538305283,0.0,360.000000000,180.000000000,\"631T\",20,5,5,5,04,00,20,03*8a1753aa\n\t", "DUALANTENNAHEADINGA,USB3,0,48.5,FINESTEERING,2107,281839.200,02000000,d426,15824;SOL_COMPUTED,NARROW_FLOAT,-1.000000000,124.470252991,58.985340118,0.0,360.000000000,180.000000000,\"631T\",20,7,7,7,04,00,20,23*a245761b\n\t", "DUALANTENNAHEADINGA,USB3,0,48.5,FINESTEERING,2107,281839.700,02000000,d426,15824;SOL_COMPUTED,NARROW_FLOAT,-1.000000000,152.317840576,70.615020752,0.0,360.000000000,180.000000000,\"631T\",18,5,5,5,04,00,20,03*7061d411\n\t", "DUALANTENNAHEADINGA,USB3,0,48.0,FINESTEERING,2107,281840.200,02000000,d426,15824;SOL_COMPUTED,L1_FLOAT,-1.000000000,81.231452942,8.750979424,0.0,360.000000000,180.000000000,\"631T\",18,6,6,3,04,00,20,01*4b849010\n\t", "DUALANTENNAHEADINGA,USB3,0,48.0,FINESTEERING,2107,281840.700,02000000,d426,15824;SOL_COMPUTED,L1_FLOAT,-1.000000000,82.520584106,5.924606323,0.0,360.000000000,180.000000000,\"631T\",18,6,6,3,04,00,20,01*b6060555\n\t", "DUALANTENNAHEADINGA,USB3,0,49.0,FINESTEERING,2107,281841.200,02000000,d426,15824;SOL_COMPUTED,L1_FLOAT,-1.000000000,85.243263245,10.185308456,0.0,360.000000000,180.000000000,\"631T\",19,6,6,3,04,00,20,01*39a33d99\n\t", "DUALANTENNAHEADINGA,USB3,0,49.0,FINESTEERING,2107,281841.700,02000000,d426,15824;SOL_COMPUTED,L1_FLOAT,-1.000000000,84.280883789,10.021371841,0.0,360.000000000,180.000000000,\"631T\",20,6,6,3,04,00,20,01*b97d95c9\n\t", "DUALANTENNAHEADINGA,USB3,0,49.5,FINESTEERING,2107,281842.200,02000000,d426,15824;SOL_COMPUTED,NARROW_FLOAT,-1.000000000,70.006813049,-31.901763916,0.0,210.151992798,180.000000000,\"631T\",17,7,7,5,04,00,20,03*5ed3d42a\n\t", "DUALANTENNAHEADINGA,USB3,0,49.5,FINESTEERING,2107,281842.700,02000000,d426,15824;SOL_COMPUTED,NARROW_FLOAT,-1.000000000,69.602676392,-30.153381348,0.0,208.420791626,180.000000000,\"631T\",17,7,7,5,04,00,20,03*0e8eebe2\n\t", "DUALANTENNAHEADINGA,USB3,0,49.5,FINESTEERING,2107,281843.200,02000000,d426,15824;SOL_COMPUTED,NARROW_FLOAT,-1.000000000,134.588546753,49.958206177,0.0,360.000000000,180.000000000,\"631T\",17,5,5,5,04,00,20,03*524a8851\n\t", "DUALANTENNAHEADINGA,USB3,0,49.5,FINESTEERING,2107,281843.700,02000000,d426,15824;SOL_COMPUTED,NARROW_FLOAT,-1.000000000,111.024063110,4.724229813,0.0,360.000000000,180.000000000,\"631T\",17,5,5,5,04,00,20,03*868053f4\n\t", "DUALANTENNAHEADINGA,USB3,0,50.0,FINESTEERING,2107,281844.200,02000000,d426,15824;SOL_COMPUTED,L1_FLOAT,-1.000000000,91.707588196,-1.773010254,0.0,360.000000000,180.000000000,\"631T\",17,6,6,3,04,00,20,01*2b557997\n\t", "DUALANTENNAHEADINGA,USB3,0,50.0,FINESTEERING,2107,281845.700,02000000,d426,15824;SOL_COMPUTED,NARROW_FLOAT,-1.000000000,48.226726532,-51.942321777,0.0,56.526073456,74.567710876,\"631T\",21,6,6,5,04,00,20,03*278cdd49\n\t", "DUALANTENNAHEADINGA,USB3,0,50.0,FINESTEERING,2107,281846.200,02000000,d426,15824;SOL_COMPUTED,L1_FLOAT,-1.000000000,98.548431396,11.085563660,0.0,360.000000000,180.000000000,\"631T\",20,6,6,3,04,00,20,01*4cd03511\n\t", "DUALANTENNAHEADINGA,USB3,0,50.0,FINESTEERING,2107,281846.700,02000000,d426,15824;SOL_COMPUTED,L1_FLOAT,-1.000000000,97.773071289,12.519289017,0.0,360.000000000,180.000000000,\"631T\",20,6,6,3,04,00,20,01*fc76e214\n\t", "DUALANTENNAHEADINGA,USB3,0,48.5,FINESTEERING,2107,281847.200,02000000,d426,15824;SOL_COMPUTED,L1_FLOAT,-1.000000000,99.566589355,2.463819742,0.0,360.000000000,180.000000000,\"631T\",20,6,6,3,04,00,20,01*aa8a8936\n\t", "DUALANTENNAHEADINGA,USB3,0,48.5,FINESTEERING,2107,281847.700,02000000,d426,15824;SOL_COMPUTED,L1_FLOAT,-1.000000000,101.704925537,-0.791503906,0.0,360.000000000,180.000000000,\"631T\",21,6,6,3,04,00,20,01*ba1d7434\n\t", "DUALANTENNAHEADINGA,USB3,0,48.0,FINESTEERING,2107,281848.200,02000000,d426,15824;SOL_COMPUTED,NARROW_FLOAT,-1.000000000,68.873619080,-13.291412354,0.0,268.060089111,180.000000000,\"631T\",21,7,7,5,04,00,20,03*0971a231\n\t", "DUALANTENNAHEADINGA,USB3,0,48.0,FINESTEERING,2107,281848.700,02000000,d426,15824;SOL_COMPUTED,NARROW_FLOAT,-1.000000000,68.326225281,-12.809478760,0.0,266.431640625,180.000000000,\"631T\",22,7,7,5,04,00,20,03*e2c6400d\n\t", "DUALANTENNAHEADINGA,USB3,0,49.0,FINESTEERING,2107,281849.200,02000000,d426,15824;SOL_COMPUTED,L1_FLOAT,-1.000000000,90.585990906,2.083147287,0.0,360.000000000,180.000000000,\"631T\",19,6,6,3,04,00,20,01*dc534f3f\n\t", "DUALANTENNAHEADINGA,USB3,0,50.5,FINESTEERING,2107,281852.700,02000000,d426,15824;SOL_COMPUTED,L1_FLOAT,-1.000000000,102.741966248,-6.929687500,0.0,360.000000000,180.000000000,\"631T\",20,6,6,3,04,00,20,01*85f8aaaa\n\t", "DUALANTENNAHEADINGA,USB3,0,48.0,FINESTEERING,2107,281853.200,02000000,d426,15824;SOL_COMPUTED,NARROW_FLOAT,-1.000000000,142.458068848,56.396076202,0.0,360.000000000,180.000000000,\"631T\",20,7,7,7,04,00,20,23*a5970788\n\t", "DUALANTENNAHEADINGA,USB3,0,48.0,FINESTEERING,2107,281853.700,02000000,d426,15824;SOL_COMPUTED,NARROW_FLOAT,-1.000000000,133.951141357,46.090900421,0.0,360.000000000,180.000000000,\"631T\",20,7,7,7,04,00,20,23*158a3a24\n\t", "INSPVAXA,USB3,0,49.5,FINESTEERING,2107,281854.250,02000000,471d,15824;INS_ALIGNMENT_COMPLETE,INS_RTKFIXED,37.37119259093,126.72297552525,7.9951,22.3000,-0.0458,0.2655,0.0156,-1.071259362,-0.181379499,98.712494459,0.4123,0.2982,0.5510,0.1098,0.0931,0.0772,0.1581,0.1591,4.8949,0f000001,0*3786ee92\n\t", "INSPVAXA,USB3,0,49.5,FINESTEERING,2107,281854.750,02000000,471d,15824;INS_ALIGNMENT_COMPLETE,INS_RTKFIXED,37.37119229237,126.72297712322,7.9984,22.3000,-0.0524,0.2443,0.0048,-0.880696017,-0.044976851,99.111895186,0.4123,0.2982,0.5510,0.1098,0.0931,0.0772,0.1581,0.1591,4.8949,0f000001,0*8e46dd5f\n\t", "DUALANTENNAHEADINGA,USB3,0,49.0,FINESTEERING,2107,281855.200,02000000,d426,15824;SOL_COMPUTED,L1_FLOAT,-1.000000000,104.180160522,-12.584655762,0.0,360.000000000,180.000000000,\"631T\",18,6,6,3,04,00,20,01*befc2b24\n\t", "DUALANTENNAHEADINGA,USB3,0,49.0,FINESTEERING,2107,281855.700,02000000,d426,15824;SOL_COMPUTED,L1_FLOAT,-1.000000000,103.651336670,-10.938995361,0.0,360.000000000,180.000000000,\"631T\",18,6,6,3,04,00,20,01*040a1ee0\n\t", "DUALANTENNAHEADINGA,USB3,0,50.0,FINESTEERING,2107,281856.200,02000000,d426,15824;SOL_COMPUTED,L1_FLOAT,-1.000000000,100.818984985,-10.711181641,0.0,360.000000000,180.000000000,\"631T\",17,6,6,3,04,00,20,01*31a96d86\n\t", "DUALANTENNAHEADINGA,USB3,0,50.0,FINESTEERING,2107,281856.700,02000000,d426,15824;SOL_COMPUTED,L1_FLOAT,-1.000000000,103.587120056,-12.575134277,0.0,360.000000000,180.000000000,\"631T\",19,6,6,3,04,00,20,01*92b9a913\n\t", "DUALANTENNAHEADINGA,USB3,0,50.5,FINESTEERING,2107,281857.200,02000000,d426,15824;SOL_COMPUTED,NARROW_FLOAT,-1.000000000,171.941314697,65.361953735,0.0,360.000000000,180.000000000,\"631T\",19,5,5,5,04,00,20,03*703cece8\n\t", "DUALANTENNAHEADINGA,USB3,0,50.5,FINESTEERING,2107,281857.700,02000000,d426,15824;SOL_COMPUTED,NARROW_FLOAT,-1.000000000,164.009658813,63.451293945,0.0,360.000000000,180.000000000,\"631T\",20,5,5,5,04,00,20,03*1783c3a5\n\t", "DUALANTENNAHEADINGA,USB3,0,46.0,FINESTEERING,2107,281865.200,02008000,d426,15824;SOL_COMPUTED,NARROW_FLOAT,-1.000000000,66.011009216,-7.448516846,0.0,202.896392822,180.000000000,\"631T\",18,7,7,5,04,00,20,03*493f8aff\n\t", "DUALANTENNAHEADINGA,USB3,0,46.0,FINESTEERING,2107,281865.700,02008000,d426,15824;SOL_COMPUTED,NARROW_FLOAT,-1.000000000,65.260665894,-8.209533691,0.0,200.108810425,180.000000000,\"631T\",19,7,7,5,04,00,20,03*eb656687\n\t", "INSPVAXA,USB3,0,47.5,FINESTEERING,2107,281866.250,02008000,471d,15824;INS_ALIGNMENT_COMPLETE,INS_RTKFIXED,37.37118340706,126.72301312751,7.9981,22.3000,-0.0652,0.2808,0.0094,-0.679665296,-0.221411969,101.808618121,0.4126,0.2985,0.5507,0.1101,0.0933,0.0772,0.1577,0.1589,4.9112,0f000001,0*dd792aaa\n\t", "DUALANTENNAHEADINGA,USB3,0,49.0,FINESTEERING,2107,281867.200,02008000,d426,15824;SOL_COMPUTED,NARROW_FLOAT,-1.000000000,93.923080444,71.863670349,0.0,360.000000000,180.000000000,\"631T\",19,5,5,5,04,00,20,03*c6afd133\n\t", "INSPVAXA,USB3,0,49.0,FINESTEERING,2107,281867.750,02008000,471d,15824;INS_ALIGNMENT_COMPLETE,INS_RTKFIXED,37.37118253054,126.72301786810,7.9941,22.3000,-0.0646,0.2786,0.0118,-0.915451137,-0.056618368,100.264591809,0.4127,0.2985,0.5509,0.1101,0.0933,0.0772,0.1576,0.1589,4.9117,0f000001,0*c2ba8d8d\n\t", "INSPVAXA,USB3,0,51.0,FINESTEERING,2107,281868.250,02000000,471d,15824;INS_ALIGNMENT_COMPLETE,INS_RTKFIXED,37.37118225307,126.72301943614,7.9928,22.3000,-0.0610,0.2887,0.0088,-0.787312923,0.119737638,100.099155235,0.4126,0.2984,0.5509,0.1099,0.0933,0.0772,0.1576,0.1589,4.9115,0f000001,0*f159e972\n\t", "INSPVAXA,USB3,0,50.5,FINESTEERING,2107,281869.250,02000000,471d,15824;INS_ALIGNMENT_COMPLETE,INS_RTKFIXED,37.37118172011,126.72302260767,7.9905,22.3000,-0.0480,0.2851,-0.0022,-0.913163720,0.118526501,100.070703566,0.4132,0.2986,0.5511,0.1100,0.0933,0.0772,0.1576,0.1589,4.9111,0f000001,0*65c3fc4b\n\t", "INSPVAXA,USB3,0,52.5,FINESTEERING,2107,281870.250,02000000,471d,15824;INS_ALIGNMENT_COMPLETE,INS_RTKFIXED,37.37118119577,126.72302574832,7.9885,22.3000,-0.0604,0.2717,0.0033,-1.019669289,-0.207037760,100.231661614,0.4136,0.2987,0.5515,0.1101,0.0932,0.0772,0.1576,0.1589,4.9104,0f000001,0*d14905d5\n\t", "INSPVAXA,USB3,0,52.5,FINESTEERING,2107,281870.750,02000000,471d,15824;INS_ALIGNMENT_COMPLETE,INS_RTKFIXED,37.37118091341,126.72302727970,7.9884,22.3000,-0.0515,0.2652,0.0073,-1.004852574,-0.259976693,100.327578359,0.4136,0.2987,0.5515,0.1101,0.0932,0.0772,0.1576,0.1589,4.9104,0f000001,0*d55530b8\n\t", "INSPVAXA,USB3,0,45.5,FINESTEERING,2107,281871.250,02000000,471d,15824;INS_ALIGNMENT_COMPLETE,INS_RTKFIXED,37.37118063962,126.72302878446,7.9883,22.3000,-0.0590,0.2793,0.0105,-0.889527092,-0.301797073,100.467035019,0.4141,0.2986,0.5519,0.1101,0.0932,0.0772,0.1576,0.1590,4.9098,0f000001,0*e8d7f1cd\n\t", "INSPVAXA,USB3,0,45.5,FINESTEERING,2107,281871.750,02000000,471d,15824;INS_ALIGNMENT_COMPLETE,INS_RTKFIXED,37.37118036572,126.72303032836,7.9872,22.3000,-0.0612,0.2876,0.0185,-0.836661662,-0.240967819,100.699833600,0.4141,0.2986,0.5519,0.1101,0.0932,0.0772,0.1576,0.1590,4.9098,0f000001,0*90542d7a\n\t", "INSPVAXA,USB3,0,47.5,FINESTEERING,2107,281872.250,02000000,471d,15824;INS_ALIGNMENT_COMPLETE,INS_RTKFIXED,37.37118005951,126.72303202791,7.9860,22.3000,-0.0539,0.2801,0.0126,-0.854711157,-0.125084871,100.880826035,0.4137,0.2986,0.5517,0.1103,0.0932,0.0772,0.1576,0.1590,4.9098,0f000001,0*60ae78ad\n\t", "INSPVAXA,USB3,0,47.5,FINESTEERING,2107,281872.750,02000000,471d,15824;INS_ALIGNMENT_COMPLETE,INS_RTKFIXED,37.37117976554,126.72303359862,7.9866,22.3000,-0.0553,0.2968,0.0085,-0.914496974,-0.073674951,101.177607301,0.4137,0.2986,0.5517,0.1103,0.0932,0.0772,0.1576,0.1590,4.9098,0f000001,0*11103b83\n\t", "INSPVAXA,USB3,0,49.5,FINESTEERING,2107,281873.250,02000000,471d,15824;INS_ALIGNMENT_COMPLETE,INS_RTKFIXED,37.37117945174,126.72303522060,7.9882,22.3000,-0.0558,0.2814,0.0151,-0.882451939,-0.080219552,101.525271935,0.4183,0.2991,0.5543,0.1109,0.0933,0.0774,0.1576,0.1591,4.9099,0f000001,0*41fa168d\n\t", "INSPVAXA,USB3,0,49.5,FINESTEERING,2107,281873.750,02000000,471d,15824;INS_ALIGNMENT_COMPLETE,INS_RTKFIXED,37.37117913037,126.72303681813,7.9893,22.3000,-0.0511,0.2800,0.0116,-0.755728696,-0.179152544,102.026561049,0.4183,0.2991,0.5543,0.1109,0.0933,0.0774,0.1576,0.1591,4.9099,0f000001,0*23029c8c\n\t", "INSPVAXA,USB3,0,50.5,FINESTEERING,2107,281874.250,02000000,471d,15824;INS_ALIGNMENT_COMPLETE,INS_RTKFIXED,37.37117879183,126.72303836597,7.9895,22.3000,-0.0480,0.2786,0.0068,-0.789121694,-0.227156967,102.683210616,0.4189,0.2989,0.5549,0.1108,0.0932,0.0774,0.1576,0.1590,4.9104,0f000001,0*be3d2619\n\t", "INSPVAXA,USB3,0,50.5,FINESTEERING,2107,281874.750,02000000,471d,15824;INS_ALIGNMENT_COMPLETE,INS_RTKFIXED,37.37117842368,126.72303989869,7.9895,22.3000,-0.0579,0.2769,0.0167,-0.872070252,-0.189275732,103.407050365,0.4189,0.2989,0.5549,0.1108,0.0932,0.0774,0.1576,0.1590,4.9104,0f000001,0*e1385384\n\t", "INSPVAXA,USB3,0,45.0,FINESTEERING,2107,281875.250,02000000,471d,15824;INS_ALIGNMENT_COMPLETE,INS_RTKFIXED,37.37117804326,126.72304144100,7.9897,22.3000,-0.0675,0.2838,0.0157,-0.838740489,-0.206654116,104.194830524,0.4175,0.2986,0.5544,0.1105,0.0931,0.0773,0.1576,0.1590,4.9111,0f000001,0*bfb33cdb\n\t", "INSPVAXA,USB3,0,45.0,FINESTEERING,2107,281875.750,02000000,471d,15824;INS_ALIGNMENT_COMPLETE,INS_RTKFIXED,37.37117766281,126.72304294804,7.9892,22.3000,-0.0643,0.2684,0.0190,-0.778611736,-0.142054720,104.951619331,0.4175,0.2986,0.5544,0.1105,0.0931,0.0773,0.1576,0.1590,4.9111,0f000001,0*c21e7554\n\t", "INSPVAXA,USB3,0,50.0,FINESTEERING,2107,281876.250,02000000,471d,15824;INS_ALIGNMENT_COMPLETE,INS_RTKFIXED,37.37117724261,126.72304445085,7.9872,22.3000,-0.0675,0.2686,0.0130,-0.693271652,-0.100470912,105.634006783,0.4157,0.2984,0.5536,0.1101,0.0930,0.0773,0.1576,0.1589,4.9121,0f000001,0*c817ed15\n\t", "INSPVAXA,USB3,0,50.0,FINESTEERING,2107,281876.750,02000000,471d,15824;INS_ALIGNMENT_COMPLETE,INS_RTKFIXED,37.37117679224,126.72304598141,7.9858,22.3000,-0.0652,0.2661,0.0195,-0.773523356,-0.163286053,106.235029610,0.4157,0.2984,0.5536,0.1101,0.0930,0.0773,0.1576,0.1589,4.9121,0f000001,0*39dfe5ae\n\t", "INSPVAXA,USB3,0,49.5,FINESTEERING,2107,281877.250,02000000,471d,15824;INS_ALIGNMENT_COMPLETE,INS_RTKFIXED,37.37117633133,126.72304748425,7.9850,22.3000,-0.0752,0.2541,0.0188,-0.756490501,-0.061250211,106.657417640,0.4141,0.2982,0.5527,0.1099,0.0930,0.0772,0.1576,0.1588,4.9134,0f000001,0*c347eea6\n\t", "INSPVAXA,USB3,0,49.5,FINESTEERING,2107,281877.750,02000000,471d,15824;INS_ALIGNMENT_COMPLETE,INS_RTKFIXED,37.37117587185,126.72304894455,7.9858,22.3000,-0.0736,0.2566,0.0182,-0.691290554,0.115671295,106.950853651,0.4141,0.2982,0.5527,0.1099,0.0930,0.0772,0.1576,0.1588,4.9134,0f000001,0*bf0681f3\n\t", "INSPVAXA,USB3,0,46.0,FINESTEERING,2107,281878.250,02000000,471d,15824;INS_ALIGNMENT_COMPLETE,INS_RTKFIXED,37.37117540642,126.72305040405,7.9858,22.3000,-0.0763,0.2617,0.0091,-0.690584467,0.289819266,107.189506996,0.4131,0.2981,0.5519,0.1099,0.0930,0.0771,0.1575,0.1588,4.9147,0f000001,0*24a15a5b\n\t", "INSPVAXA,USB3,0,46.0,FINESTEERING,2107,281878.750,02000000,471d,15824;INS_ALIGNMENT_COMPLETE,INS_RTKFIXED,37.37117493552,126.72305185756,7.9850,22.3000,-0.0783,0.2561,0.0099,-0.645148551,0.263210480,107.376836106,0.4131,0.2981,0.5519,0.1099,0.0930,0.0771,0.1575,0.1588,4.9147,0f000001,0*d1c1fe45\n\t", "INSPVAXA,USB3,0,48.5,FINESTEERING,2107,281879.250,02000000,471d,15824;INS_ALIGNMENT_COMPLETE,INS_RTKFIXED,37.37117447448,126.72305323836,7.9839,22.3000,-0.0805,0.2449,0.0028,-0.594473310,0.228947195,107.558540148,0.4129,0.2981,0.5511,0.1100,0.0931,0.0771,0.1575,0.1588,4.9163,0f000001,0*ee394e1f\n\t", "INSPVAXA,USB3,0,48.5,FINESTEERING,2107,281879.750,02000000,471d,15824;INS_ALIGNMENT_COMPLETE,INS_RTKFIXED,37.37117397984,126.72305472755,7.9828,22.3000,-0.0867,0.2510,0.0095,-0.498608617,0.229834885,107.620298376,
